vi "formatTimestamp.vi"(9 "Value":timestamp, 11 "StringFormatter":refnum<class "StringFormatter.lvclass">) -> (1 "Formatted Value":string)   [LabVIEW 2013, in "OpenStringFormatter.lvlib" / "StringFormatter.lvclass"]
uses:
  StringFormatter.lvclass
  StringFormatter.lvclass/StringFormatter.ctl
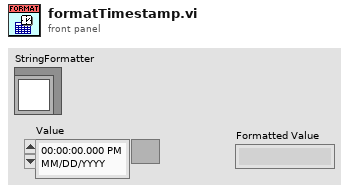
[diagram p1: front panel]
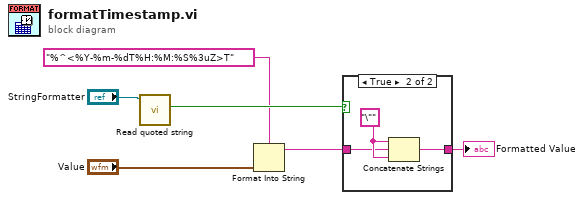
[diagram p0: block diagram]
diagram:
  n1 = call "Read quoted string.vi"("StringFormatter in"="StringFormatter") -> ("quoted string"=w6:bool)  [unwired: 9 in, 1 out]
  n2 = Format Into String(format string="%^<%Y-%m-%dT%H:%M:%S%3uZ>T", "Value") -> (resulting string=w2:string)  [unwired: 2 in, 1 out]
  n3 = case shown="True" w6 {
    tunnel: [w7 w9] -> w4
    tunnel: w2 -> [w7 w8]
    frame False {
    }
    frame True {
      w10 = "\"" ("string")
      n4 = Concatenate Strings(w10, w8, w10) -> (w9:string)
    }
  }
  "Formatted Value" <- w4
